vi "fibonacci.vi"() -> ()   [LabVIEW 2020]
panel:
  out "Array":i32[](array[numeric])
  in  "Numeric":i32
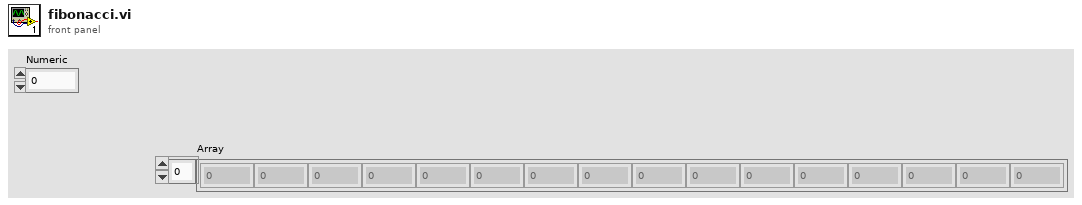
[diagram p1: front panel]
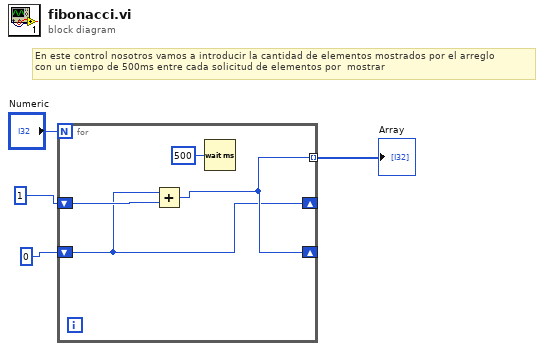
[diagram p0: block diagram]
diagram:
  # "En este control nosotros vamos a introducir la cantidad de elementos mostrados por el arreglo \ncon un tiempo de 500ms entre cada solicitud de elementos por  mostrar"
  n1 = for {
    N: "Numeric" -> [_]
    shift-right: [w6] -> _
    shift-left: 1 -> [w8]
    shift-right: [w7] -> _
    shift-left: 0 -> [w6]
    tunnel: [w7] -> w1 mode=indexing
    n2 = Add(x=w6, y=w8) -> (x+y=w7:i32)
    n3 = Wait (ms)(milliseconds to wait=u32 500) -> ()  [unwired: 1 out]
  }
  "Array" <- w1
